vi "Hide Module.vi"(8 "error in":errorcluster) -> (0 "error out":errorcluster)   [LabVIEW 2014, in "Events Lib.lvlib"]
uses:
  Events Lib.lvlib
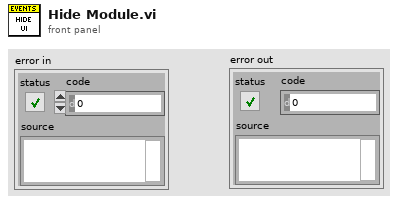
[diagram p1: front panel]
types:
  T1 = enum16{"Create Events", "Get Events", "Destroy Events"}
  T2 = typedef "Events Lib.lvlib/Events TypeDef.ctl" = cluster{"Stop Event":refnum<user-event>, "Chart Send Value":refnum<user-event>, "Show Module":refnum<user-event>, "Hide Module":refnum<user-event>}
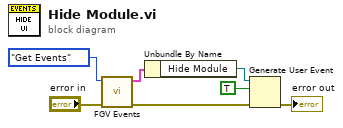
[diagram p0: block diagram]
diagram:
  n1 = call "FGV Events.vi"("error in"="error in", "Action"=T1."Get Events") -> ("error out"=w3:errorcluster, "Cluster"=w5:T2)  [unwired: 8 in]
  n2 = Unbundle By Name(w5) -> ("Hide Module"=w4:refnum<user-event>)
  n3 = Generate User Event(user event=w4, event data cluster=TRUE, error in=w3) -> (error out=→"error out":errorcluster)  [unwired: 1 in, 1 out]
